vi "Crop Graph.vi"(8 "error in":errorcluster, 11 "Image In":i32[][](array[numeric])) -> (0 "error out":errorcluster, 2 "Invert Roi":bool[](array[boolean]), 3 "Roi":T1)   [LabVIEW 2023]
uses:
  <vilib>/Utility/miscctls.llb/LVPoint32TypeDef.ctl
  queue/Front Panel Message Queue.lvlib
panel:
  out "Image Roi":i32[][](graph)
  out "Table Out":i32[][](array[numeric])
  in  "inY":bool
  in  "inX":bool
  in  "point":enum16{"-", "bottom - left", "top - right"}(ring)
  in  "crop":bool
  out "Image Roi Out":i32[][](graph)
  in  "reset":bool
  in  "type":enum16{"linear", "square", "log"}(ring)
  out "element":i32
  in  "Stop":bool
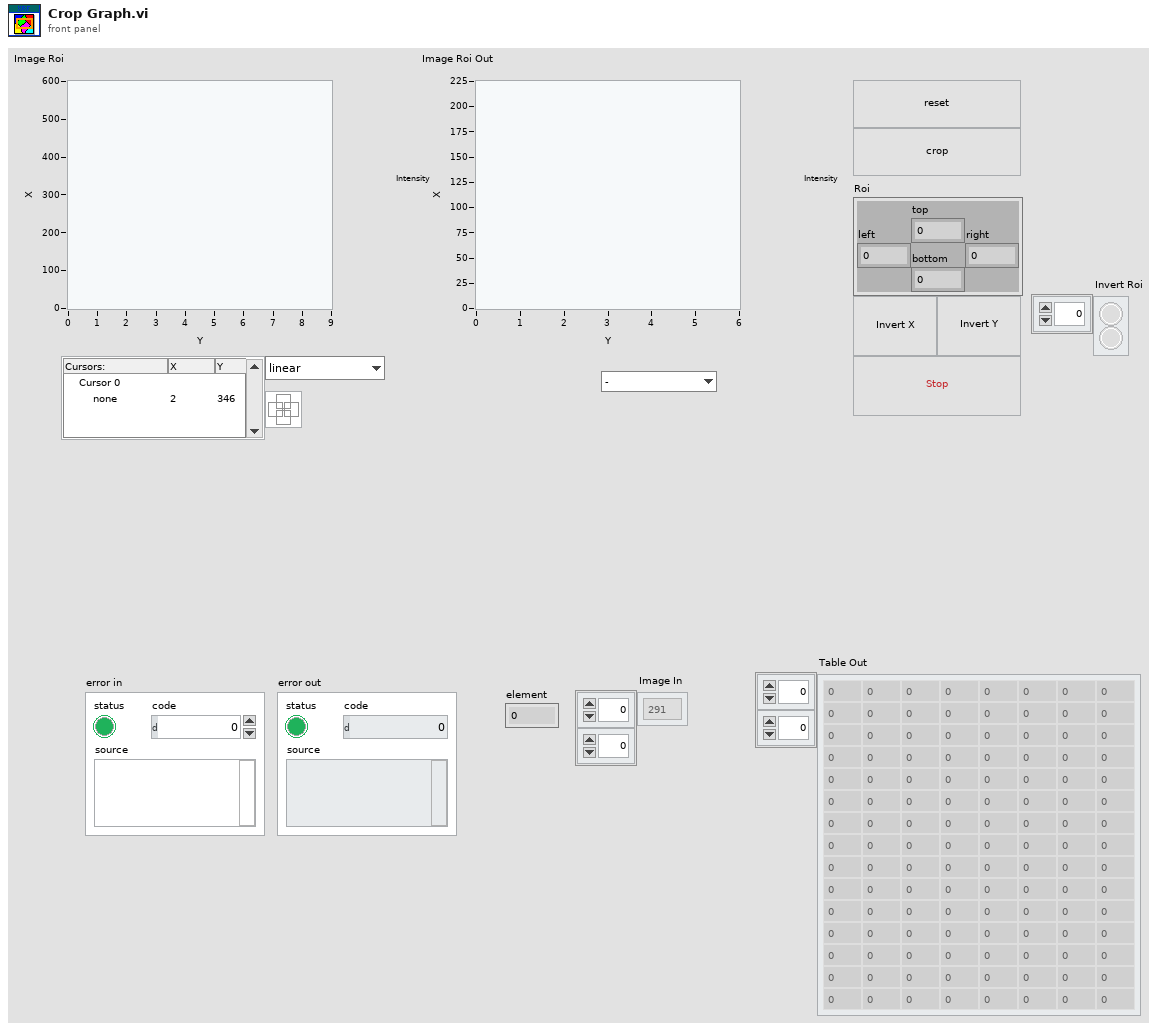
[diagram p1: front panel]
types:
  T1 = cluster{"left":i16, "top":i16, "right":i16, "bottom":i16}
  T2 = typedef "Front Panel Message Queue.lvlib/load Message Queues.ctl" = cluster{"Main":refnum<queue>}
  T3 = typedef "LVPoint32TypeDef.ctl" = cluster{"Horizontal":i32, "Vertical":i32}
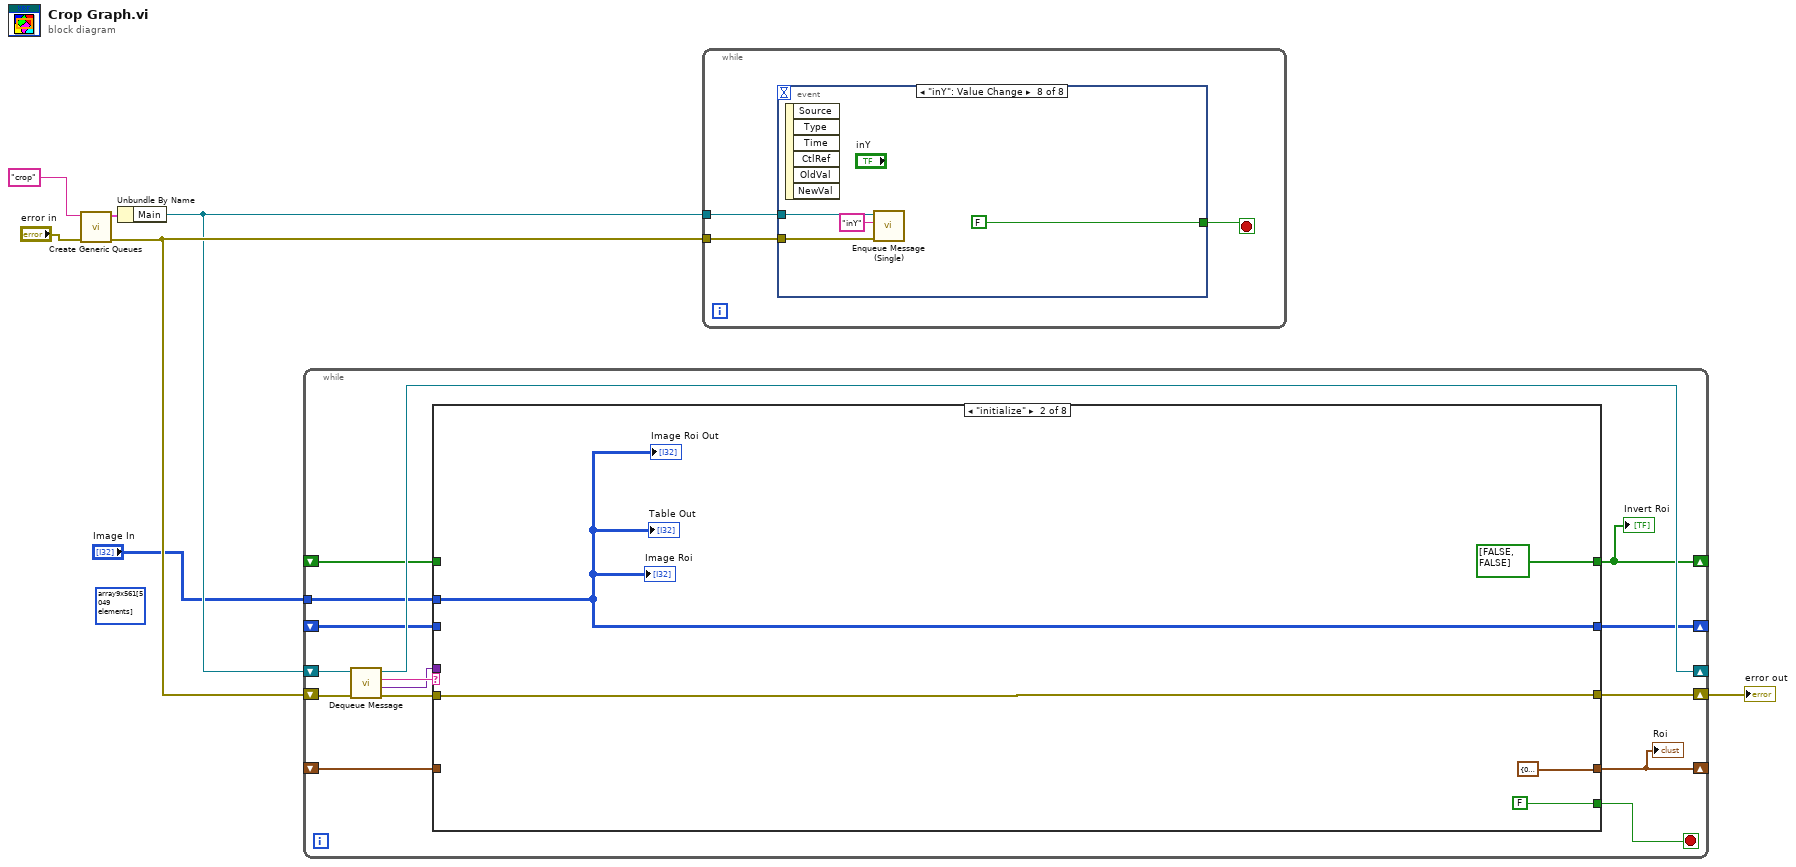
[diagram p0: block diagram]
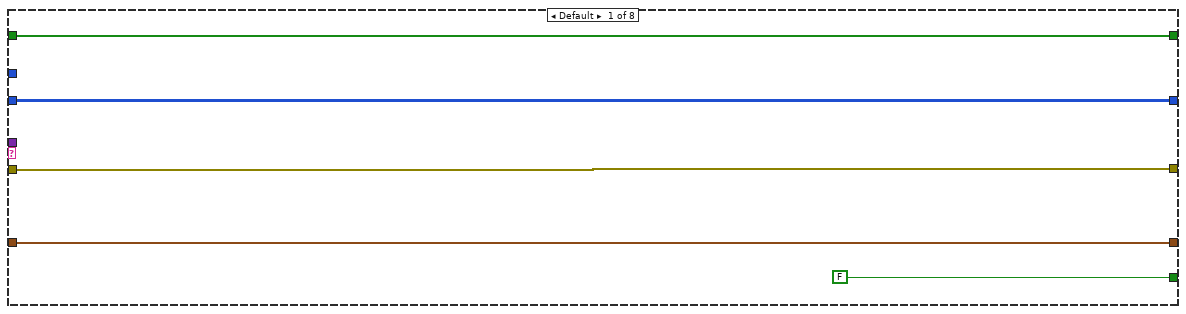
[diagram p2: hidden frame]
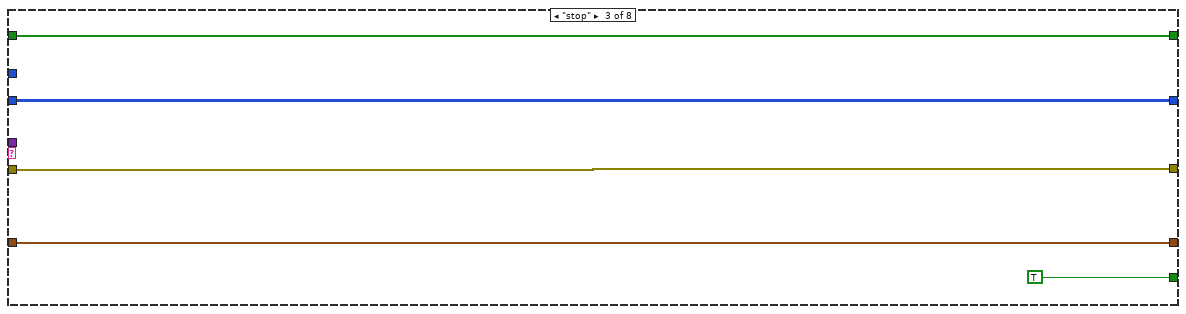
[diagram p3: hidden frame]
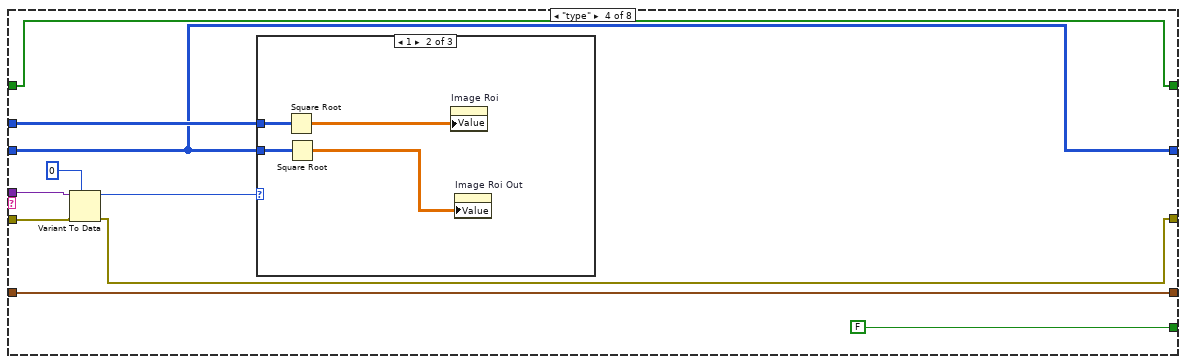
[diagram p4: hidden frame]
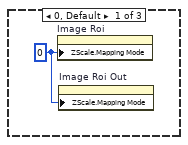
[diagram p5: hidden frame]
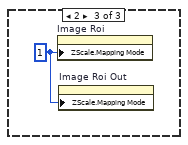
[diagram p6: hidden frame]
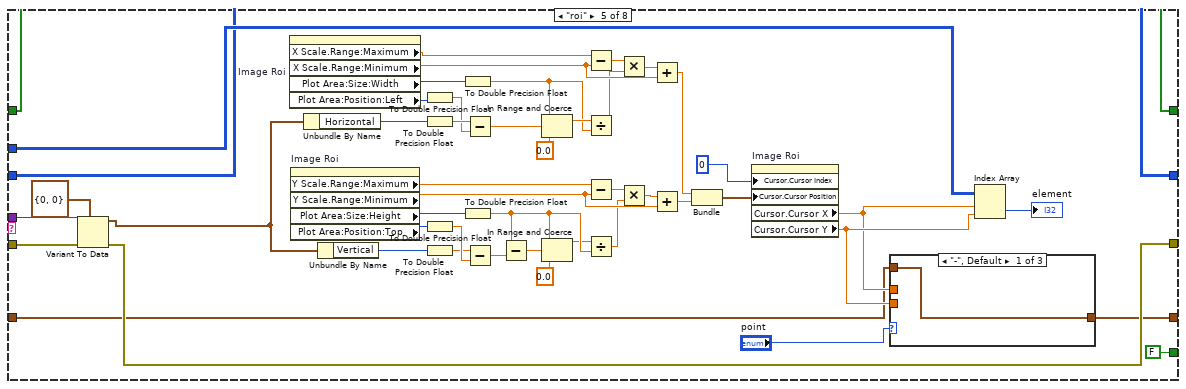
[diagram p7: hidden frame]
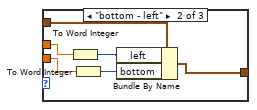
[diagram p8: hidden frame]
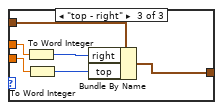
[diagram p9: hidden frame]
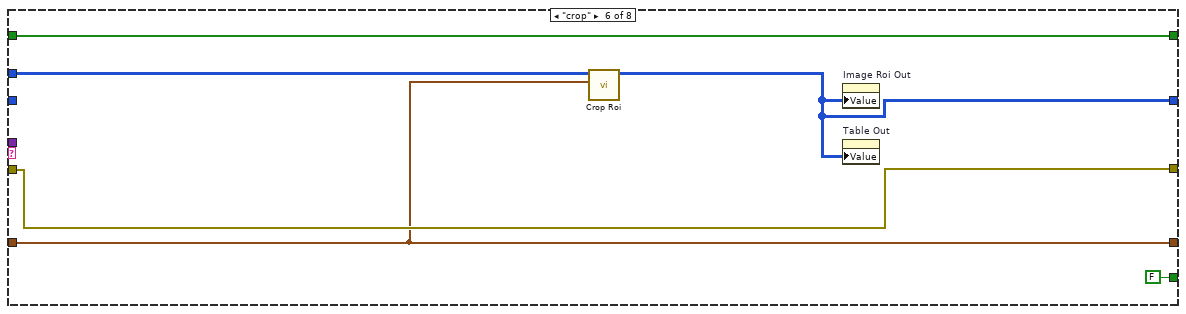
[diagram p10: hidden frame]
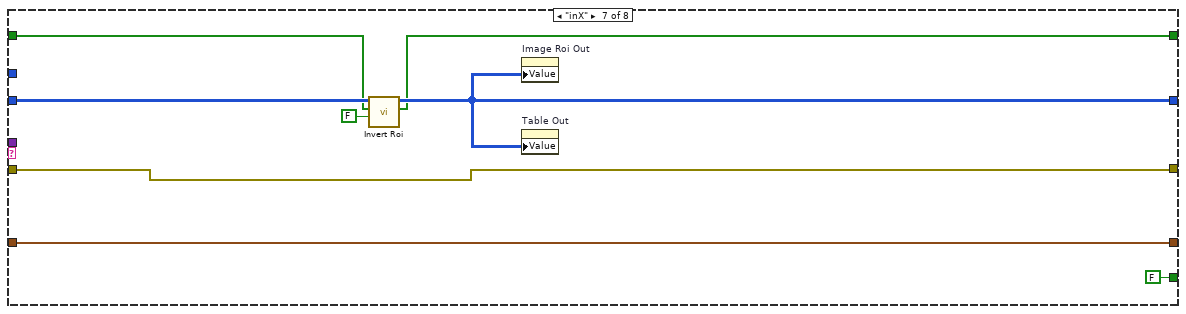
[diagram p11: hidden frame]
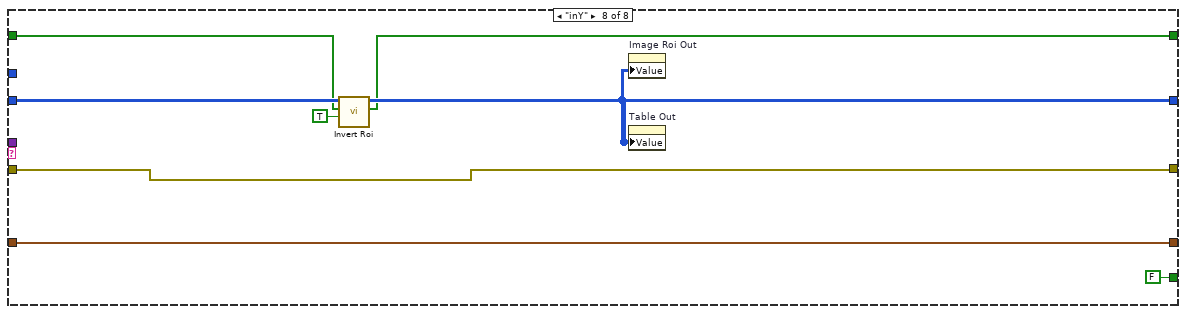
[diagram p12: hidden frame]
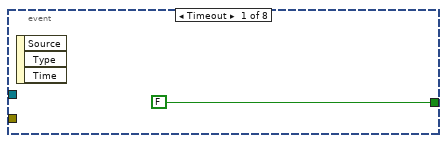
[diagram p13: hidden frame]
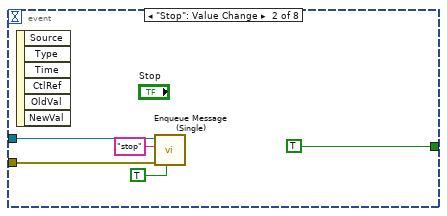
[diagram p14: hidden frame]
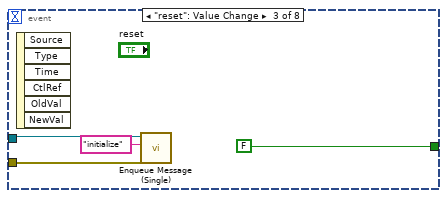
[diagram p15: hidden frame]
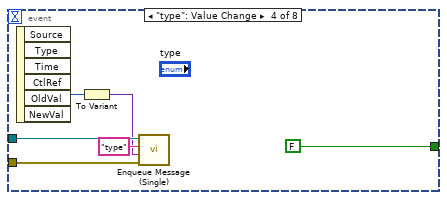
[diagram p16: hidden frame]
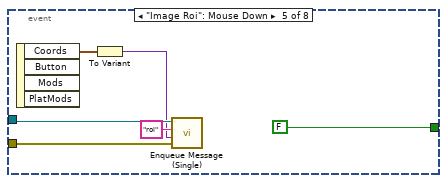
[diagram p17: hidden frame]
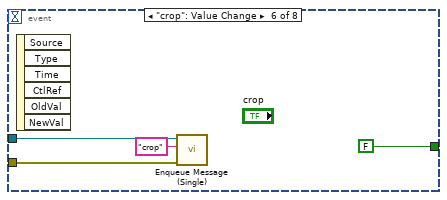
[diagram p18: hidden frame]
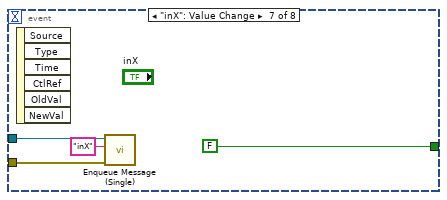
[diagram p19: hidden frame]
diagram:
  (unwired) i32[][] array9x561[5049 elements] ("Image Roi")
  n1 = call "Create Generic Queues.vi"("error in (no error)"="error in", "name"="crop") -> ("error out"=w4:errorcluster, "Message Queues"=w5:T2)  [unwired: 8 in]
  n2 = Unbundle By Name(w5) -> ("Main"=w3:refnum<queue>)
  n3 = while {
    shift-right: [w17] -> w2
    shift-left: w4 -> [w22]
    shift-right: [w20] -> _
    shift-left: w3 -> [w21]
    shift-right: [w12] -> _
    shift-left: _ -> [w15]
    shift-right: [w11] -> _
    shift-left: _ -> [w10]
    tunnel: "Image In" -> [w13]
    shift-right: [w9] -> _
    shift-left: _ -> [w8]
    stop <- w16 stop-if-true
    n4 = call "Dequeue Message.vi"("error in (no error)"=w22, "Message Queue"=w21) -> ("error out"=w19:errorcluster, "Message Data"=w14:variant, "Message"=w18:string, "dup Message Queue"=w20:refnum<queue>)  [unwired: 5 in, 1 out]
    n5 = case shown="\"initialize\"" w18 {
      tunnel: w19 -> [w27 w32 w36 w45 w100 w119 w128 w136]
      tunnel: [w27 w32 w36 w44 w62 w119 w128 w136] -> w17
      tunnel: [FALSE FALSE TRUE FALSE FALSE FALSE FALSE FALSE] -> w16
      tunnel: [w25 T1 {"left"=0, "top"=0, "right"=0, "bottom"=0} ("rect") w35 w46 w56 w118 w127 w135] -> w12
      tunnel: w15 -> [w25 _ w35 w46 w57 w118 w127 w135]
      tunnel: w14 -> [_ _ _ w43 w101 _ _ _]
      tunnel: w13 -> [_ w29 _ w40 w59 w117 _ _]
      tunnel: [w24 w29 w34 w39 w55 w116 w123 w133] -> w11
      tunnel: w10 -> [w24 _ w34 w39 w55 _ w124 w132]
      tunnel: [w23 bool[] [FALSE, FALSE] ("Invert Roi") w33 w38 w54 w115 w121 w129] -> w9
      tunnel: w8 -> [w23 _ w33 w38 w54 w115 w122 w130]
      frame Default {
      }
      frame "initialize" {
        "Image Roi Out" <- w29
        "Table Out" <- w29
        "Image Roi" <- w29
      }
      frame "stop" {
      }
      frame "type" {
        n6 = Variant To Data(error in=w45, type=u16 0, Variant=w43) -> (data=w41:u16, error out=w44:errorcluster)
        n7 = case shown="1" w41 {
          tunnel: w40 -> [_ w52 _]
          tunnel: w39 -> [_ w50 _]
          frame 0, Default {
            w48 = u8 0 ("Z Scale.Mapping Mode")
            n8 = property on="Image Roi" class="IntGraph (strict)"("ZScale.Mapping Mode"=w48) -> ()  [unwired: 2 in, 2 out]
            n9 = property on="Image Roi Out" class="IntGraph (strict)"("ZScale.Mapping Mode"=w48) -> ()  [unwired: 2 in, 2 out]
          }
          frame 1 {
            n10 = Square Root(x=w52) -> (sqrt(x)=w51:dbl[][])
            n11 = Square Root(x=w50) -> (sqrt(x)=w49:dbl[][])
            n12 = property on="Image Roi" class="IntGraph (strict)"("Value"=w51) -> ()  [unwired: 2 in, 2 out]
            n13 = property on="Image Roi Out" class="IntGraph (strict)"("Value"=w49) -> ()  [unwired: 2 in, 2 out]
          }
          frame 2 {
            w53 = u8 1 ("Z Scale.Mapping Mode")
            n14 = property on="Image Roi" class="IntGraph (strict)"("ZScale.Mapping Mode"=w53) -> ()  [unwired: 2 in, 2 out]
            n15 = property on="Image Roi Out" class="IntGraph (strict)"("ZScale.Mapping Mode"=w53) -> ()  [unwired: 2 in, 2 out]
          }
        }
      }
      frame "roi" {
        n16 = Variant To Data(error in=w100, type=T3 {"Horizontal"=0, "Vertical"=0} ("Coords"), Variant=w101) -> (data=w58:T3, error out=w62:errorcluster)
        n17 = property on="Image Roi" class="IntensityGraph (strict)"() -> ("X Scale.Range:Maximum"=w89:dbl, "X Scale.Range:Minimum"=w90:dbl, "Plot Area:Size:Width"=w91:u32, "Plot Area:Position:Left"=w92:i32)  [unwired: 2 in, 2 out]
        n18 = property on="Image Roi" class="IntensityGraph (strict)"() -> ("Y Scale.Range:Maximum"=w65:dbl, "Y Scale.Range:Minimum"=w70:dbl, "Plot Area:Size:Height"=w73:u32, "Plot Area:Position:Top"=w80:i32)  [unwired: 2 in, 2 out]
        n19 = Unbundle By Name(w58) -> ("Horizontal"=w93:i32)
        n20 = Unbundle By Name(w58) -> ("Vertical"=w66:i32)
        n21 = To Double Precision Float(number=w92) -> (double precision float=w84:dbl)
        n22 = To Double Precision Float(number=w93) -> (double precision float=w85:dbl)
        n23 = To Double Precision Float(number=w80) -> (double precision float=w75:dbl)
        n24 = To Double Precision Float(number=w66) -> (double precision float=w74:dbl)
        n25 = To Double Precision Float(number=w91) -> (double precision float=w81:dbl)
        n26 = To Double Precision Float(number=w73) -> (double precision float=w79:dbl)
        n27 = Subtract(x=w85, y=w84) -> (x-y=w96:dbl)
        n28 = Subtract(x=w74, y=w75) -> (x-y=w72:dbl)
        n29 = Subtract(x=w79, y=w72) -> (x-y=w76:dbl)
        n30 = In Range and Coerce(upper limit=w81, x=w96, lower limit=0.0) -> (coerced(x)=w82:dbl)  [unwired: 1 out]
        n31 = In Range and Coerce(upper limit=w79, x=w76, lower limit=0.0) -> (coerced(x)=w78:dbl)  [unwired: 1 out]
        n32 = Subtract(x=w89, y=w90) -> (x-y=w88:dbl)
        n33 = Divide(x=w82, y=w81) -> (x/y=w87:dbl)
        n34 = Subtract(x=w65, y=w70) -> (x-y=w67:dbl)
        n35 = Divide(x=w78, y=w79) -> (x/y=w68:dbl)
        n36 = Multiply(x=w88, y=w87) -> (x*y=w86:dbl)
        n37 = Multiply(x=w67, y=w68) -> (x*y=w69:dbl)
        n38 = Add(x=w86, y=w90) -> (x+y=w94:dbl)
        n39 = Add(x=w69, y=w70) -> (x+y=w71:dbl)
        n40 = Bundle(w94, w71) -> (w95:cluster{dbl, dbl})  [unwired: 1 in]
        n41 = property on="Image Roi" class="IntGraph (strict)"("Cursor.Cursor Index"=0, "Cursor.Cursor Position"=w95) -> ("Cursor.Cursor X"=w97:dbl, "Cursor.Cursor Y"=w98:dbl)  [unwired: 2 in, 2 out]
        n42 = case shown="\"-\", Default" "point" {
          tunnel: w97 -> [_ w107 w113]
          tunnel: w57 -> [w102 w108 w114]
          tunnel: w98 -> [_ w106 w110]
          tunnel: [w102 w105 w112] -> w56
          frame "-", Default {
          }
          frame "bottom - left" {
            n43 = To Word Integer(number=w107) -> (16bit integer=w104:i16)
            n44 = To Word Integer(number=w106) -> (16bit integer=w103:i16)
            n45 = Bundle By Name(cluster=w108, "left"=w104, "bottom"=w103) -> (w105:T1)
          }
          frame "top - right" {
            n46 = To Word Integer(number=w113) -> (16bit integer=w111:i16)
            n47 = To Word Integer(number=w110) -> (16bit integer=w109:i16)
            n48 = Bundle By Name(cluster=w114, "right"=w111, "top"=w109) -> (w112:T1)
          }
        }
        n49 = Index Array(array=w59, index (row)=w97, index (col)=w98) -> (element=→"element":i32)
      }
      frame "crop" {
        n50 = call "Crop Roi.vi"("Roi"=w118, "Table Roi In"=w117) -> ("Table Roi Out"=w116:i32[][])  [unwired: 9 in]
        n51 = property on="Image Roi Out" class="IntGraph (strict)"("Value"=w116) -> ()  [unwired: 2 in, 2 out]
        n52 = property on="Table Out" class="Arr (strict)"("Value"=w116) -> ()  [unwired: 2 in, 2 out]
      }
      frame "inX" {
        n53 = call "Invert Roi.vi"("Invert Columns?"=FALSE, "Invert Roi In"=w122, "Table Roi In"=w124) -> ("Invert Roi Out"=w121:bool[], "Table Roi Out"=w123:i32[][])  [unwired: 7 in]
        n54 = property on="Image Roi Out" class="IntGraph (strict)"("Value"=w123) -> ()  [unwired: 2 in, 2 out]
        n55 = property on="Table Out" class="Arr (strict)"("Value"=w123) -> ()  [unwired: 2 in, 2 out]
      }
      frame "inY" {
        n56 = call "Invert Roi.vi"("Invert Columns?"=TRUE, "Invert Roi In"=w130, "Table Roi In"=w132) -> ("Invert Roi Out"=w129:bool[], "Table Roi Out"=w133:i32[][])  [unwired: 7 in]
        n57 = property on="Image Roi Out" class="IntGraph (strict)"("Value"=w133) -> ()  [unwired: 2 in, 2 out]
        n58 = property on="Table Out" class="Arr (strict)"("Value"=w133) -> ()  [unwired: 2 in, 2 out]
      }
    }
    "Roi" <- w12
    "Invert Roi" <- w9
  }
  "error out" <- w2
  n59 = while {
    tunnel: w4 -> [w138]
    tunnel: w3 -> [w137]
    stop <- w139 stop-if-true
    n60 = event shown="[7] \"inY\": Value Change" {
      selector: _ -> [_ _ _ _ _ _ _ _]
      dyn-events: _ -> [_ _ _ _ _ _ _ _]
      timeout: _ -> [_ _ _ _ _ _ _ _]
      tunnel: [FALSE ("Stop") TRUE ("Stop") FALSE ("Stop") FALSE ("Stop") FALSE ("Stop") FALSE ("Stop") FALSE ("Stop") FALSE ("Stop")] -> w139
      tunnel: w138 -> [_ w144 w148 w154 w160 w164 w167 w171]
      tunnel: w137 -> [_ w143 w147 w153 w159 w163 w168 w172]
      event Timeout {
        n61 = event-data() -> ()  [unwired: 1 in, 3 out]
      }
      event "Stop": Value Change {
        n62 = event-data() -> ()  [unwired: 1 in, 6 out]
        n63 = call "Enqueue Message (Single).vi"("Priority Message? (F)"=TRUE, "error in (no error)"=w144, "Message"="stop", "Message Queue"=w143) -> ()  [unwired: 6 in, 2 out]
      }
      event "reset": Value Change {
        n64 = event-data() -> ()  [unwired: 1 in, 6 out]
        n65 = call "Enqueue Message (Single).vi"("error in (no error)"=w148, "Message"="initialize", "Message Queue"=w147) -> ()  [unwired: 7 in, 2 out]
      }
      event "type": Value Change {
        n66 = event-data() -> ("NewVal"=w151:enum16{"linear", "square", "log"})  [unwired: 1 in, 5 out]
        n67 = To Variant(anything=w151) -> (Variant=w150:variant)
        n68 = call "Enqueue Message (Single).vi"("error in (no error)"=w154, "Message Data"=w150, "Message"="type", "Message Queue"=w153) -> ()  [unwired: 6 in, 2 out]
      }
      event "Image Roi": Mouse Down {
        n69 = event-data() -> ("Coords"=w157:T3)  [unwired: 1 in, 3 out]
        n70 = To Variant(anything=w157) -> (Variant=w156:variant)
        n71 = call "Enqueue Message (Single).vi"("error in (no error)"=w160, "Message Data"=w156, "Message"="roi", "Message Queue"=w159) -> ()  [unwired: 6 in, 2 out]
      }
      event "crop": Value Change {
        n72 = event-data() -> ()  [unwired: 1 in, 6 out]
        n73 = call "Enqueue Message (Single).vi"("error in (no error)"=w164, "Message"="crop", "Message Queue"=w163) -> ()  [unwired: 7 in, 2 out]
      }
      event "inX": Value Change {
        n74 = event-data() -> ()  [unwired: 1 in, 6 out]
        n75 = call "Enqueue Message (Single).vi"("error in (no error)"=w167, "Message"="inX", "Message Queue"=w168) -> ()  [unwired: 7 in, 2 out]
      }
      event "inY": Value Change {
        n76 = event-data() -> ()  [unwired: 1 in, 6 out]
        n77 = call "Enqueue Message (Single).vi"("error in (no error)"=w171, "Message"="inY", "Message Queue"=w172) -> ()  [unwired: 7 in, 2 out]
      }
    }
  }
